vi "Get Bool.vi"(7 "Optional":bool, 8 "error in (no error)":errorcluster, 9 "Default":bool, 10 "Name":string, 11 "LV Argument Parser in":refnum<class "LV Argument Parser.lvclass">) -> (0 "error out":errorcluster, 1 "Value":bool, 2 "key not found?":bool, 3 "LV Argument Parser out":refnum<class "LV Argument Parser.lvclass">)   [LabVIEW 2020, in "LV ArgParse.lvlib" / "LV Argument Parser.lvclass"]
uses:
  LV Argument Parser.lvclass
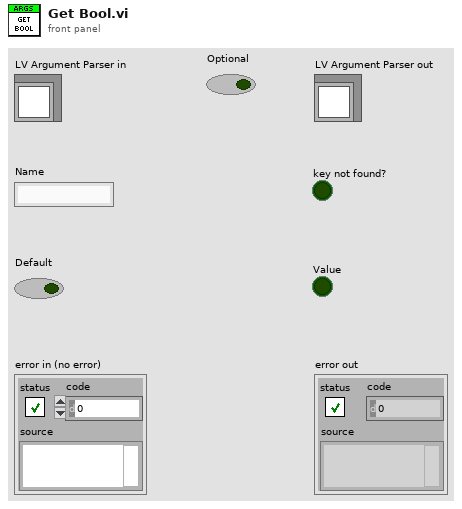
[diagram p1: front panel]
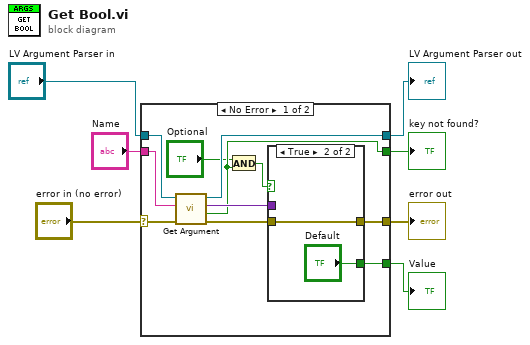
[diagram p0: block diagram]
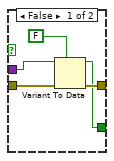
[diagram p2: hidden frame]
diagram:
  n1 = case shown="No Error" "error in (no error)" {
    selector: "error in (no error)" -> [w18 w27]
    tunnel: [w13 w27] -> w6
    tunnel: [w15 w26] -> w4
    tunnel: "LV Argument Parser in" -> [w16 w26]
    tunnel: "Name" -> [w14 _]
    tunnel: [w10 _] -> w2
    tunnel: [w11 _] -> w1
    frame No Error {
      n2 = call "Get Argument.vi"("error in (no error)"=w18, "Name"=w14, "LV Argument Parser in"=w16) -> ("error out"=w17:errorcluster, "key not found?"=w10:bool, "element"=w12:variant, "LV Argument Parser out"=w15:refnum<class "LV Argument Parser.lvclass">)  [unwired: 5 in]
      n3 = And(x="Optional", y=w10) -> (x .and. y?=w9:bool)
      n4 = case shown="True" w9 {
        tunnel: w17 -> [w23 w25]
        tunnel: [w22 w25] -> w13
        tunnel: w12 -> [w21 _]
        tunnel: [w19 "Default"] -> w11
        frame False {
          n5 = Variant To Data(error in=w23, type=FALSE, Variant=w21) -> (data=w19:bool, error out=w22:errorcluster)
        }
        frame True {
        }
      }
    }
    frame Error {
    }
  }
  "error out" <- w6
  "LV Argument Parser out" <- w4
  "key not found?" <- w2
  "Value" <- w1
